vi "Get Cache.vi"(11 "Framework in":refnum<class "Framework.lvclass">) -> (2 "Cache":refnum<class "Cache.lvclass">, 3 "Framework out":refnum<class "Framework.lvclass">)   [LabVIEW 2017]
uses:
  Framework.lvclass
  Cache/Cache.lvclass
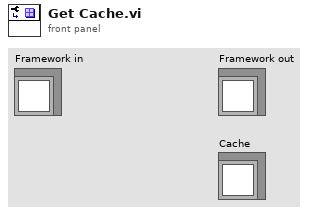
[diagram p1: front panel]
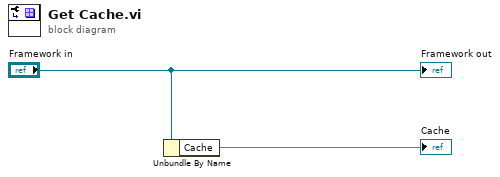
[diagram p0: block diagram]
diagram:
  n1 = Unbundle By Name("Framework in") -> ("Cache"=→"Cache")
  "Framework out" <- "Framework in"
